vi "config Spark Max.vi"(5 "Reverse Limit switch":T1=enum."Normally Closed", 6 "LIMIT SW\nEnabled?":bool, 7 "Forward Limit switch":T1=enum."Normally Closed", 8 "error in (no error)":errorcluster, 11 "motor\ndefaults":T2={"description"="", "MOTOR SELECT"=0, "Installed?"=FALSE, "CAN ID"=0, "refnum name"="", "Invert"=FALSE, "Idle Mode"=enum."Coast", "Current limiting"={"Linearized"=FALSE, "Free Speed (A)"=0.0, "Primay (A)"=0.0, "Limit RPM (0)"=0}, "MOTOR PIDF coefficients"={"PIDF"={"P Gain"=0.001, "I Gain"=0.0, "D Gain"=0.0, "F Gain"=0.0012, "I Zone"=0.0, "Min Output"=-1.0, "Max Output"=1.0}, "Smart Motion"={"Max Velocity"=1900.0, "Max Acceleration"=750.0, "Minimum Velocity Output"=0.1, "Allowed Closed Loop Error"=0.02}}, "gear ratio"=0.0} {"gear ratio" format="%_5f"; "MOTOR SELECT" items=["REV NEO"=5676, "REV NEO 550"=11000, "VEX Falcon"=6380, "WC Kraken"=6000]}) -> (0 "error out":errorcluster, 3 "MotorControlDevRef":T8)   [LabVIEW 2023]
uses:
  <vilib>/Rock Robotics/WPI/MotorControl/WPI_MotorControlDeviceRef.ctl
  <vilib>/Rock Robotics/WPI/MotorControl/WPI_MotorControlType.ctl
  <vilib>/Rock Robotics/SystemInterfaces/DIO/FPGA_DIOPWMChannel.ctl
  <vilib>/Rock Robotics/WPI/PWM/WPI_PWMDeadband.ctl
  <vilib>/Rock Robotics/SystemInterfaces/DIO/FPGA_DIOChannel.ctl
  ctrl defs/ctrl swerve motor.ctl
  ctrl defs/ctrl MOTOR SELECT.ctl
  <vilib>/Rock Robotics/WPI/ThirdParty/REV Robotics/REVLib/Typedef/Spark MAX Idle Mode.ctl
  ctrl defs/ctrl Spark MAX current limiting.ctl
  ctrl defs/ctrl motor PIDF coefficients.ctl
  <vilib>/Rock Robotics/WPI/ThirdParty/REV Robotics/REVLib/Typedef/Spark MAX Smart Motion Parameters.ctl
  <vilib>/Rock Robotics/WPI/ThirdParty/REV Robotics/REVLib/Typedef/Spark MAX Limit Switch Polarity.ctl
  <vilib>/Rock Robotics/WPI/ThirdParty/REV Robotics/REVLib/Typedef/SPARK Closed Loop Slot.ctl
  <vilib>/Rock Robotics/WPI/ThirdParty/REV Robotics/REVLib/SubVI/Public/SPARK Open Brushless.vi
  <vilib>/Rock Robotics/WPI/ThirdParty/REV Robotics/REVLib/SubVI/Public/SPARK Configure Basic Inverted.vi
  <vilib>/Rock Robotics/WPI/ThirdParty/REV Robotics/REVLib/SubVI/Public/SPARK Configure Basic Idle Mode.vi
  <vilib>/Rock Robotics/WPI/ThirdParty/REV Robotics/REVLib/SubVI/Public/SPARK Configure Basic Ramp Rate.vi
  <vilib>/Rock Robotics/WPI/ThirdParty/REV Robotics/REVLib/SubVI/Public/SPARK Configure Absolute Encoder Conversion Factors.vi
  <vilib>/Rock Robotics/WPI/ThirdParty/REV Robotics/REVLib/SubVI/Public/SPARK Configure Limit Switch Forward.vi
  <vilib>/Rock Robotics/WPI/ThirdParty/REV Robotics/REVLib/SubVI/Public/SPARK Configure Limit Switch Reverse.vi
  <vilib>/Rock Robotics/WPI/ThirdParty/REV Robotics/REVLib/SubVI/Public/SPARK Configure Closed Loop Smart Motion.vi
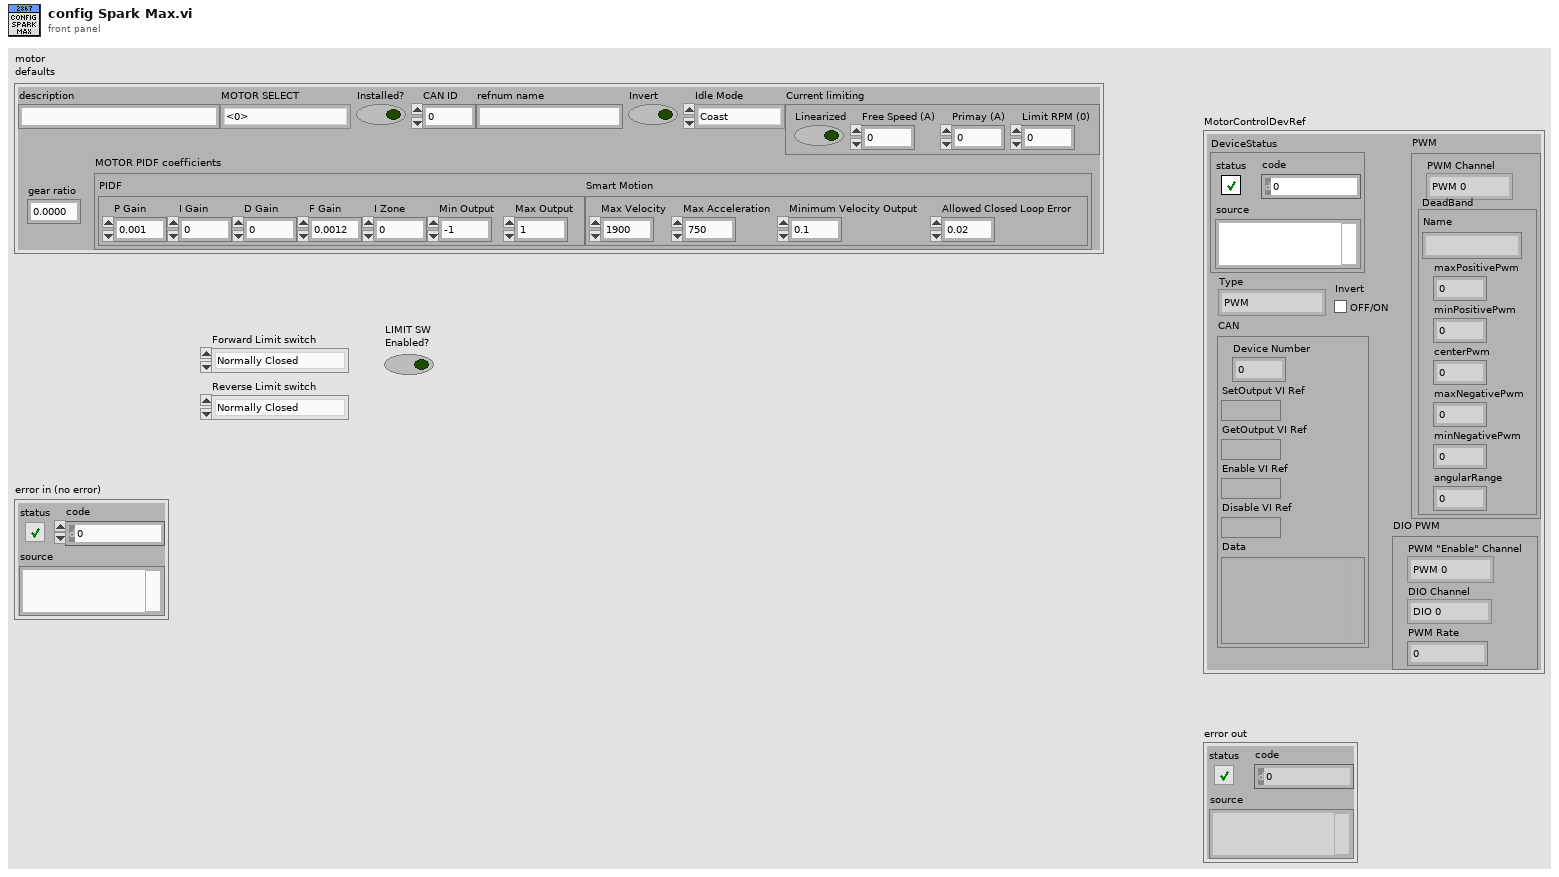
[diagram p1: front panel]
types:
  T1 = typedef "Spark MAX Limit Switch Polarity.ctl" = enum16{"Normally Open", "Normally Closed"}
  T2 = typedef "ctrl swerve motor.ctl" = cluster{"description":string, "MOTOR SELECT":T3, "Installed?":bool, "CAN ID":u8, "refnum name":string, "Invert":bool, "Idle Mode":T4, "Current limiting":T5, "MOTOR PIDF coefficients":T6, "gear ratio":dbl}
  T3 = typedef "ctrl MOTOR SELECT.ctl" = i16
  T4 = typedef "Spark MAX Idle Mode.ctl" = enum16{"Coast", "Brake"}
  T5 = typedef "ctrl Spark MAX current limiting.ctl" = cluster{"Linearized":bool, "Free Speed (A)":dbl, "Primay (A)":dbl, "Limit RPM (0)":u32}
  T6 = typedef "ctrl motor PIDF coefficients.ctl" = cluster{"PIDF":cluster{"P Gain":dbl, "I Gain":dbl, "D Gain":dbl, "F Gain":dbl, "I Zone":dbl, "Min Output":dbl, "Max Output":dbl}, "Smart Motion":T7}
  T7 = typedef "Spark MAX Smart Motion Parameters.ctl" = cluster{"Max Velocity":dbl, "Max Acceleration":dbl, "Minimum Velocity Output":dbl, "Allowed Closed Loop Error":dbl}
  T8 = typedef "WPI_MotorControlDeviceRef.ctl" = cluster{"DeviceStatus":errorcluster, "Type":T9, "PWM":cluster{"PWM Channel":T10, "DeadBand":T11}, "CAN":cluster{"Device Number":u8, "SetOutput VI Ref":variant, "GetOutput VI Ref":variant, "Enable VI Ref":variant, "Disable VI Ref":variant, "Data":variant}, "Invert":bool, "DIO PWM":cluster{"PWM \"Enable\" Channel":T10, "DIOChannel":T12, "PWM Rate":dbl}}
  T9 = typedef "WPI_MotorControlType.ctl" = enum16{"PWM", "CAN", "DIO PWM"}
  T10 = typedef "FPGA_DIOPWMChannel.ctl" = enum8{"PWM 0", "PWM 1", "PWM 2", "PWM 3", "PWM 4", "PWM 5", "PWM 6", "PWM 7", "PWM 8", "PWM 9", "PWM MXP 0", "PWM MXP 1", "PWM MXP 2", "PWM MXP 3", "PWM MXP 4", "PWM MXP 5", "PWM MXP 6", "PWM MXP 7", "PWM MXP 8", "PWM MXP 9", "Invalid"}
  T11 = typedef "WPI_PWMDeadband.ctl" = cluster{"Name":string, "maxPositivePwm":i32, "minPositivePwm":i32, "centerPwm":i32, "maxNegativePwm":i32, "minNegativePwm":i32, "angularRange":u16}
  T12 = typedef "FPGA_DIOChannel.ctl" = enum8{"DIO 0", "DIO 1", "DIO 2", "DIO 3", "DIO 4", "DIO 5", "DIO 6", "DIO 7", "DIO 8", "DIO 9", "DIO MXP 0", "DIO MXP 1", "DIO MXP 2", "DIO MXP 3", "DIO MXP 4", "DIO MXP 5", "DIO MXP 6", "DIO MXP 7", "DIO MXP 8", "DIO MXP 9", "DIO MXP 10", "DIO MXP 11", "DIO MXP 12", "DIO MXP 13", "DIO MXP 14", "DIO MXP 15", "SPI Port CS1", "SPI Port CS2", "SPI Port CS3", "SPI Port MISO", "SPI Port MOSI", "Invalid"}
  T13 = typedef "SPARK Closed Loop Slot.ctl" = u16
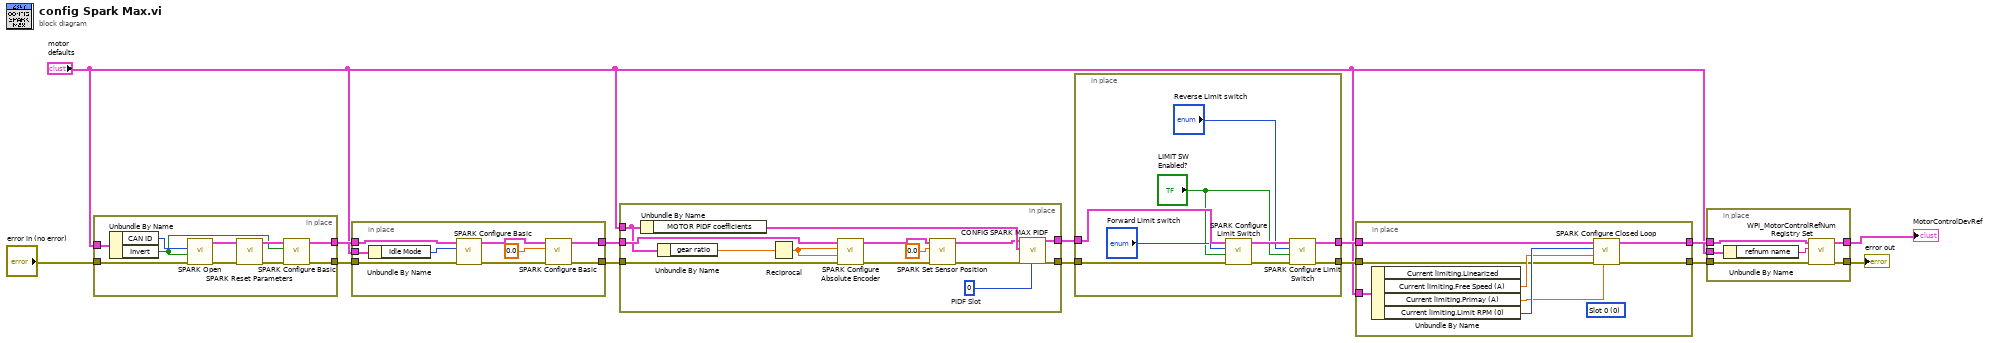
[diagram p0: block diagram]
diagram:
  n1 = in-place {
    in-place-border: [w23] -> w10
    in-place-border: [w22] -> w9
    in-place-border: "motor\ndefaults" -> [w19]
    in-place-border: "error in (no error)" -> [w15]
    n2 = Unbundle By Name(w19) -> ("CAN ID"=w24:u8, "Invert"=w16:bool)
    n3 = call-poly <vilib>:"SPARK Open.vi"("error in (no error)"=w15, "Invert"=w16, "Device Number"=w24) -> ("error out"=w20:errorcluster, "MotorControlDeviceRef"=w21:T8)  [unwired: 7 in]
    n4 = call <vilib>:"SPARK Reset Parameters.vi"("error in"=w20, "MotorControlDeviceRef"=w21) -> ("error out"=w17:errorcluster, "MotorControlDeviceRef"=w18:T8)  [unwired: 8 in]
    n5 = call-poly <vilib>:"SPARK Configure Basic.vi"("error in (no error)"=w17, "Inverted (F)"=w16, "MotorControlDeviceRef in"=w18) -> ("error out"=w23:errorcluster, "MotorControlDeviceRef out"=w22:T8)  [unwired: 7 in]
  }
  n6 = in-place {
    in-place-border: w10 -> [w33]
    in-place-border: w9 -> [w32]
    in-place-border: [w28] -> w5
    in-place-border: [w26] -> w6
    in-place-border: "motor\ndefaults" -> [w29]
    n7 = Unbundle By Name(w29) -> ("Idle Mode"=w30:T4)
    n8 = call-poly <vilib>:"SPARK Configure Basic.vi"("error in (no error)"=w33, "Idle Mode"=w30, "MotorControlDeviceRef in"=w32) -> ("error out"=w27:errorcluster, "MotorControlDeviceRef out"=w31:T8)  [unwired: 7 in]
    n9 = call-poly <vilib>:"SPARK Configure Basic.vi"("error in (no error)"=w27, "Seconds from neutral to full (0)"=sgl 0.0, "MotorControlDeviceRef in"=w31) -> ("error out"=w26:errorcluster, "MotorControlDeviceRef"=w28:T8)  [unwired: 7 in]
  }
  n10 = in-place {
    in-place-border: w6 -> [w47]
    in-place-border: w5 -> [w46]
    in-place-border: [w42] -> w4
    in-place-border: [w41] -> w3
    in-place-border: "motor\ndefaults" -> [w40]
    w38 = 0  # PIDF Slot
    n11 = Unbundle By Name(w40) -> ("MOTOR PIDF coefficients"=w39:T6)
    n12 = Unbundle By Name(w40) -> ("gear ratio"=w45:dbl)
    n13 = Reciprocal(x=w45) -> (1/x=w44:dbl)
    n14 = call-poly <vilib>:"SPARK Configure Absolute Encoder.vi"("error in (no error)"=w47, "Velocity Conversion Factor"=w44, "Position Conversion Factor"=w44, "MotorControlDeviceRef in"=w46) -> ("error out"=w35:errorcluster, "MotorControlDeviceRef out"=w43:T8)  [unwired: 6 in]
    n15 = call <vilib>:"SPARK Set Sensor Position.vi"("error in"=w35, "Position"=0.0, "MotorControlDeviceRef"=w43) -> ("error out"=w34:errorcluster, "MotorControlDeviceRef"=w37:T8)  [unwired: 7 in]
    n16 = call "CONFIG SPARK MAX PIDF.vi"("MotorControlDevRef"=w37, "MOTOR PIDF coefficients"=w39, "error in (no error)"=w34, "PIDF Slot"=w38) -> ("MotorControlDevRef OUT"=w42:T8, "error out"=w41:errorcluster)  [unwired: 14 in]
  }
  n17 = in-place {
    in-place-border: w4 -> [w56]
    in-place-border: [w54] -> w8
    in-place-border: w3 -> [w52]
    in-place-border: [w50] -> w7
    n18 = call-poly <vilib>:"SPARK Configure Limit Switch.vi"("error in"=w52, "Enabled? (T)"="LIMIT SW\nEnabled?", "Polarity (Normally Open)"="Forward Limit switch", "MotorControlDeviceRef in"=w56) -> ("error out"=w51:errorcluster, "MotorControlDeviceRef out"=w55:T8)  [unwired: 6 in]
    n19 = call-poly <vilib>:"SPARK Configure Limit Switch.vi"("error in"=w51, "Enabled? (T)"="LIMIT SW\nEnabled?", "Polarity (Normally Open)"="Reverse Limit switch", "MotorControlDeviceRef in"=w55) -> ("error out"=w50:errorcluster, "MotorControlDeviceRef out"=w54:T8)  [unwired: 6 in]
  }
  n20 = in-place {
    in-place-border: [w64] -> w13
    in-place-border: [w60] -> w11
    in-place-border: w8 -> [w59]
    in-place-border: w7 -> [w58]
    in-place-border: "motor\ndefaults" -> [w57]
    (unwired) T13 0 items=["Slot 0", "Slot 1", "Slot 2", "Slot 3"] ("Closed Loop Slot (0)")
    n21 = Unbundle By Name(w57) -> ("Current limiting.Free Speed (A)"=w62:dbl, "Current limiting.Primay (A)"=w61:dbl, "Current limiting.Limit RPM (0)"=w63:u32)  [unwired: 1 out]
    n22 = call-poly <vilib>:"SPARK Configure Closed Loop.vi"("Closed Loop Slot (0)"=w61, "error in"=w58, "Max Acceleration"=w62, "Max Velocity"=w63, "MotorControlDeviceRef in"=w59) -> ("error out"=w64:errorcluster, "MotorControlDeviceRef out"=w60:T8)  [unwired: 5 in]
  }
  n23 = in-place {
    in-place-border: [w70] -> w14
    in-place-border: w13 -> [w69]
    in-place-border: [w68] -> w12
    in-place-border: w11 -> [w67]
    in-place-border: "motor\ndefaults" -> [w65]
    n24 = Unbundle By Name(w65) -> ("refnum name"=w66:string)
    n25 = call <vilib>:"WPI_MotorControlRefNum Registry Set.vi"("error in (no error)"=w69, "refnum name"=w66, "MotorControlDevRef"=w67) -> ("error out"=w70:errorcluster, "MotorControlDevRef"=w68:T8)  [unwired: 7 in]
  }
  "error out" <- w14
  "MotorControlDevRef" <- w12
